vi "MeasurementService GetMetadata.vi"(6 "contextId":T1, 8 "error in":errorcluster, 9 "timeout (ms)":i32=-1, 10 "Request Data":T12, 11 "gRPC ID":T1) -> (0 "error out":errorcluster, 2 "Response Data":T2, 3 "gRPC ID out":T1)   [LabVIEW 2021, in "Measurement Service Client.lvlib"]
uses:
  Measurement Service Client.lvlib
  14035477-4c25-4107-8ed5-d0c4ef420ce5.vi
  RPC Messages/ni_measurementlink_measurement_v2_MeasurementDetails_Flat.ctl
  RPC Messages/google_protobuf_Field_Kind.ctl
  RPC Messages/ni_measurementlink_measurement_v2_ConfigurationParameter_AnnotationsEntry_Flat.ctl
  RPC Messages/ni_measurementlink_measurement_v2_ConfigurationParameter_Flat.ctl
  RPC Messages/google_protobuf_Any_Flat.ctl
  RPC Messages/ni_measurementlink_measurement_v2_Output_AnnotationsEntry_Flat.ctl
  RPC Messages/ni_measurementlink_measurement_v2_Output_Flat.ctl
  RPC Messages/ni_measurementlink_measurement_v2_MeasurementSignature_Flat.ctl
  RPC Messages/ni_measurementlink_measurement_v2_UserInterfaceDetails_Flat.ctl
  RPC Messages/ni_measurementlink_measurement_v2_GetMetadataResponse_Flat.ctl
  <vilib>/gRPC/LabVIEW gRPC Library/Shared/grpcId.ctl
  <vilib>/gRPC/LabVIEW gRPC Library/grpc-lvsupport-release.lvlib
  RPC Messages/ni_measurementlink_measurement_v2_UserInterfaceDetails.ctl
  RPC Messages/ni_measurementlink_measurement_v2_Output_AnnotationsEntry.ctl
  RPC Messages/ni_measurementlink_measurement_v2_Output.ctl
  RPC Messages/google_protobuf_Any.ctl
  RPC Messages/ni_measurementlink_measurement_v2_ConfigurationParameter_AnnotationsEntry.ctl
  RPC Messages/ni_measurementlink_measurement_v2_ConfigurationParameter.ctl
  RPC Messages/ni_measurementlink_measurement_v2_MeasurementSignature.ctl
  RPC Messages/ni_measurementlink_measurement_v2_MeasurementDetails.ctl
  RPC Messages/ni_measurementlink_measurement_v2_GetMetadataResponse.ctl
  RPC Messages/ni_measurementlink_measurement_v2_GetMetadataRequest.ctl
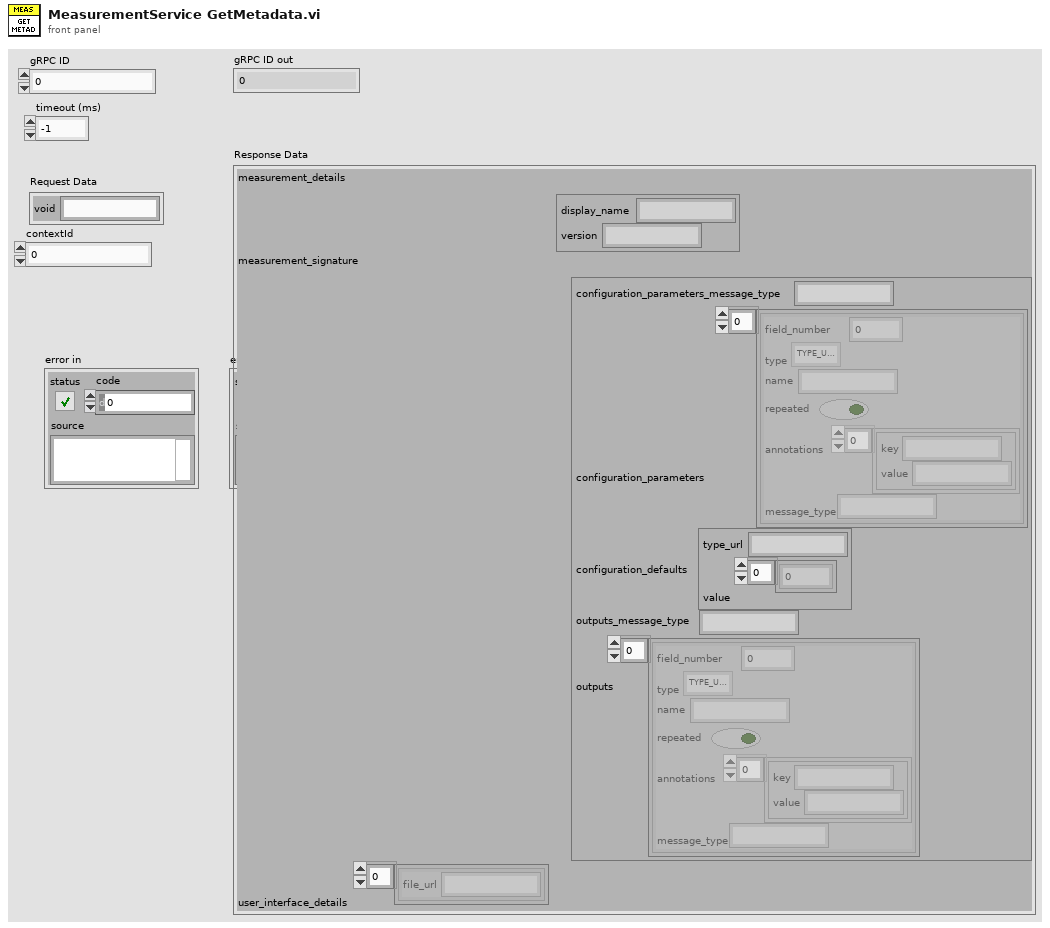
[diagram p1: front panel]
types:
  T1 = typedef "grpc-lvsupport-release.lvlib/grpcId.ctl" = u64
  T2 = typedef "Measurement Service Client.lvlib/ni_measurementlink_measurement_v2_GetMetadataResponse.ctl" = cluster{"measurement_details":T3, "measurement_signature":T4, "user_interface_details":T11[]}
  T3 = typedef "Measurement Service Client.lvlib/ni_measurementlink_measurement_v2_MeasurementDetails.ctl" = cluster{"display_name":string, "version":string}
  T4 = typedef "Measurement Service Client.lvlib/ni_measurementlink_measurement_v2_MeasurementSignature.ctl" = cluster{"configuration_parameters_message_type":string, "configuration_parameters":T5[], "configuration_defaults":T8, "outputs_message_type":string, "outputs":T9[]}
  T5 = typedef "Measurement Service Client.lvlib/ni_measurementlink_measurement_v2_ConfigurationParameter.ctl" = cluster{"field_number":i32, "type":T6, "name":string, "repeated":bool, "annotations":T7[], "message_type":string}
  T6 = typedef "Measurement Service Client.lvlib/google_protobuf_Field_Kind.ctl" = enum32{"TYPE_UNKNOWN", "TYPE_DOUBLE", "TYPE_FLOAT", "TYPE_INT64", "TYPE_UINT64", "TYPE_INT32", "TYPE_FIXED64", "TYPE_FIXED32", "TYPE_BOOL", "TYPE_STRING", "TYPE_GROUP", "TYPE_MESSAGE", "TYPE_BYTES", "TYPE_UINT32", "TYPE_ENUM", "TYPE_SFIXED32", "TYPE_SFIXED64", "TYPE_SINT32", "TYPE_SINT64"}
  T7 = typedef "Measurement Service Client.lvlib/ni_measurementlink_measurement_v2_ConfigurationParameter_AnnotationsEntry.ctl" = cluster{"key":string, "value":string}
  T8 = typedef "Measurement Service Client.lvlib/google_protobuf_Any.ctl" = cluster{"type_url":string, "value":u8[]}
  T9 = typedef "Measurement Service Client.lvlib/ni_measurementlink_measurement_v2_Output.ctl" = cluster{"field_number":i32, "type":T6, "name":string, "repeated":bool, "annotations":T10[], "message_type":string}
  T10 = typedef "Measurement Service Client.lvlib/ni_measurementlink_measurement_v2_Output_AnnotationsEntry.ctl" = cluster{"key":string, "value":string}
  T11 = typedef "Measurement Service Client.lvlib/ni_measurementlink_measurement_v2_UserInterfaceDetails.ctl" = cluster{"file_url":string}
  T12 = typedef "Measurement Service Client.lvlib/ni_measurementlink_measurement_v2_GetMetadataRequest.ctl" = cluster{"void":string}
  T13 = typedef "Measurement Service Client.lvlib/ni_measurementlink_measurement_v2_GetMetadataResponse_Flat.ctl" = cluster{"measurement_details":T14, "measurement_signature":T15, "user_interface_details":T21[]}
  T14 = typedef "Measurement Service Client.lvlib/ni_measurementlink_measurement_v2_MeasurementDetails_Flat.ctl" = cluster{"display_name":string, "version":string}
  T15 = typedef "Measurement Service Client.lvlib/ni_measurementlink_measurement_v2_MeasurementSignature_Flat.ctl" = cluster{"configuration_parameters_message_type":string, "configuration_parameters":T16[], "configuration_defaults":T18, "outputs_message_type":string, "outputs":T19[]}
  T16 = typedef "Measurement Service Client.lvlib/ni_measurementlink_measurement_v2_ConfigurationParameter_Flat.ctl" = cluster{"field_number":i32, "type":T6, "name":string, "repeated":bool, "annotations":T17[], "message_type":string}
  T17 = typedef "Measurement Service Client.lvlib/ni_measurementlink_measurement_v2_ConfigurationParameter_AnnotationsEntry_Flat.ctl" = cluster{"key":string, "value":string}
  T18 = typedef "Measurement Service Client.lvlib/google_protobuf_Any_Flat.ctl" = cluster{"type_url":string, "value":u8[]}
  T19 = typedef "Measurement Service Client.lvlib/ni_measurementlink_measurement_v2_Output_Flat.ctl" = cluster{"field_number":i32, "type":T6, "name":string, "repeated":bool, "annotations":T20[], "message_type":string}
  T20 = typedef "Measurement Service Client.lvlib/ni_measurementlink_measurement_v2_Output_AnnotationsEntry_Flat.ctl" = cluster{"key":string, "value":string}
  T21 = typedef "Measurement Service Client.lvlib/ni_measurementlink_measurement_v2_UserInterfaceDetails_Flat.ctl" = cluster{"file_url":string}
  T22 = typedef "ni.measurementlink.measurement.v2.api.lvlib/Measurement Service Client.lvlib/ni_measurementlink_measurement_v2_GetMetadataRequest_Flat.ctl" = cluster{"void":string}
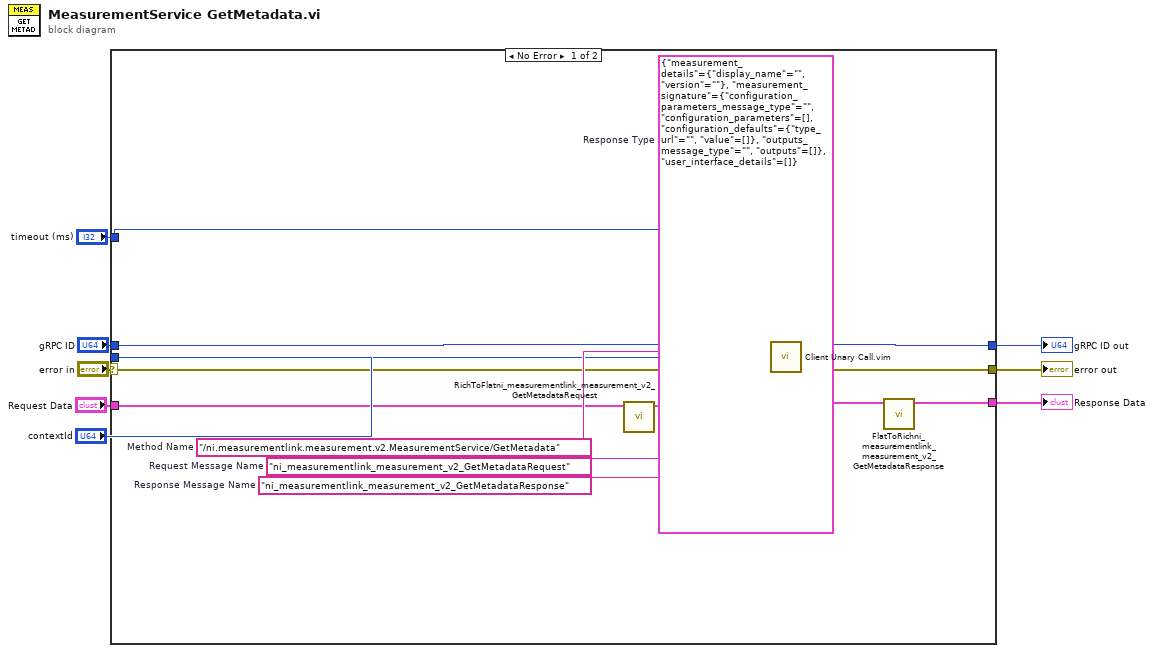
[diagram p0: block diagram]
diagram:
  n1 = case shown="No Error" "error in" {
    selector: "error in" -> [w18 w23]
    tunnel: [w17 w23] -> w7
    tunnel: "gRPC ID" -> [w16 w24]
    tunnel: [w15 w24] -> w5
    tunnel: "Request Data" -> [w12 _]
    tunnel: [w9 _] -> w3
    tunnel: "timeout (ms)" -> [w14 _]
    tunnel: "contextId" -> [w13 _]
    frame No Error {
      w19 = "ni_measurementlink_measurement_v2_GetMetadataResponse"  # Response Message Name
      w20 = "ni_measurementlink_measurement_v2_GetMetadataRequest"  # Request Message Name
      w21 = T13 {"measurement_details"={"display_name"="", "version"=""}, "measurement_signature"={"configuration_parameters_message_type"="", "configuration_parameters"=[], "configuration_defaults"={"type_url"="", "value"=[]}, "outputs_message_type"="", "outputs"=[]}, "user_interface_details"=[]}  # Response Type
      w22 = "/ni.measurementlink.measurement.v2.MeasurementService/GetMetadata"  # Method Name
      n2 = call "RichToFlatni_measurementlink_measurement_v2_GetMetadataRequest.vi"("InputCluster"=w12) -> ("OutputCluster"=w11:T22)  [unwired: 10 in]
      n3 = call "Client Unary Call.vim"("ClientID in"=w16, "Response Type"=w21, "timeout (ms)"=w14, "Method Name"=w22, "contextId"=w13, "Request Data"=w11, "error in"=w18, "Request Message Name"=w20, "Response Message Name"=w19) -> ("ClientID out"=w15:u64, "Response Data"=w10:T13, "error out"=w17:errorcluster)  [unwired: 4 in]
      n4 = call "FlatToRichni_measurementlink_measurement_v2_GetMetadataResponse.vi"("InputCluster"=w10) -> ("OutputCluster"=w9:T2)  [unwired: 10 in]
    }
    frame Error {
    }
  }
  "error out" <- w7
  "gRPC ID out" <- w5
  "Response Data" <- w3
